vi "Create From Variant.vi"(8 "error in (no error)":errorcluster, 10 "Variant":variant, 11 "JSON Datatype in":refnum<class "JSON Null.lvclass">) -> (0 "error out":errorcluster, 3 "JSON Datatype out":refnum<class "JSON Null.lvclass">)   [LabVIEW 2016, in "LVJSON.lvlib" / "JSON Null.lvclass"]
doc: "Creates a new JSON instance from the given Variant."
uses:
  JSON Null.lvclass
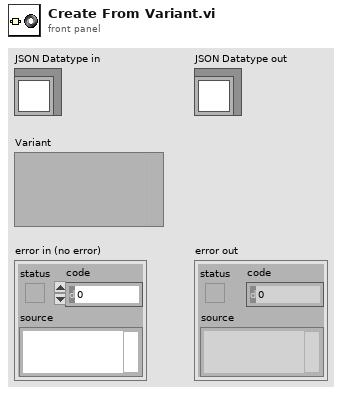
[diagram p1: front panel]
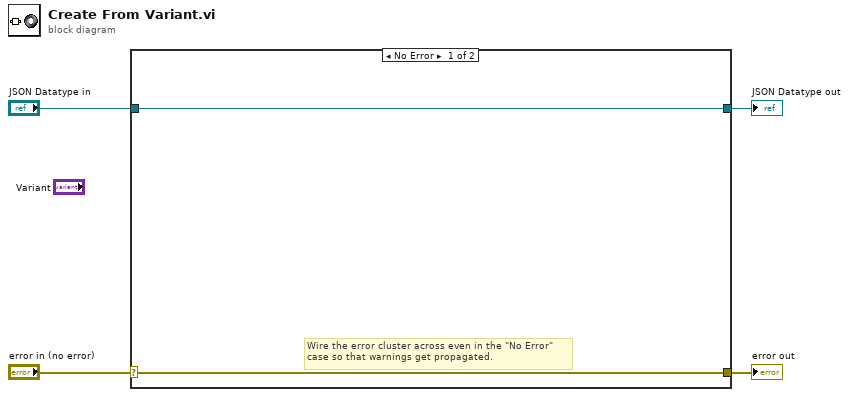
[diagram p0: block diagram]
diagram:
  n1 = case shown="No Error" "error in (no error)" {
    selector: "error in (no error)" -> [w5 w8]
    tunnel: [w5 w8] -> w3
    tunnel: [w6 w7] -> w1
    tunnel: "JSON Datatype in" -> [w6 w7]
    frame No Error {
      # "Wire the error cluster across even in the \"No Error\"\ncase so that warnings get propagated."
    }
    frame Error {
    }
  }
  "error out" <- w3
  "JSON Datatype out" <- w1
